vi "Test Panel - Multiple Loops.vi"(7 "Sequence Loop Settings":T4={"Number of Loops"=1, "Delay Between Loops"=0.5} {"Delay Between Loops" format="%#_6ps"}, 8 "Error in":errorcluster, 9 "TDMS Name Mapping":T6={"FGEN Channel Mapping"=[["0", "Chn0"]], "DAQ Channel Mapping"=[["port0/line1", "PA ON"], ["port0/line2", "Gate IN"], ["port0/line3", "Damping"], ["port0/line4", "Rx ON"]], "FGEN Wfm List"=[["Wfm1", "FGEN_Wfm1"], ["Wfm2", "FGEN_Wfm2"]], "DAQ Wfm List"=[["Wfm1", "DAQ_Wfm1"], ["Wfm2", "DAQ_Wfm2"]]}, 10 "Wavefom Sequence":T5={"FGEN Wfm Sequence"=["Wfm1"], "DAQ Wfm Sequence"=["Wfm1"], "Loops"=[1]}, 11 "Resource Settings":T3={"FGEN Resource"="", "DAQmx Resource"="", "TDMS File Path"=path "", "Scope Resource"="", "Scope Config File Path"=path "", "Trigger Delay"=0.0, "Duration"=-1.0, "Fetch Timeout"=5.0} {"Fetch Timeout" format="%#.5ps"; "Duration" format="%#_6ps"; "Trigger Delay" format="%#_gs"}) -> (0 "Error out":errorcluster, 1 "FFT Waveforms (dB)":T8(graph), 2 "FFT Waveforms (Volt RMS)":T8(graph), 3 "Time Domain Waveforms":T8(graph), 4 "All Results Ctrl Refs":T10, 5 "Average FFT (dB)":T8(graph))   [LabVIEW 2025]
uses:
  Live Graph Plotter/Live Graph Plotter.lvclass
  <extravilib>/ChannelInstances/Tag-bool.lvlib
  Typedef/Scope Result Ctrl Refs.ctl
  Typedef/TDMS Name Mapping.ctl
  Typedef/Resource Settings.ctl
panel:
  out "Actual Sample Rates":T1 {"FGEN Sample Rate" format="%#_6pHz"; "DAQ Sample Rate" format="%#_6pHz"; "SCOPE Sample Rate" format="%#_6pHz"}
  in  "Stop":bool
  in  "Tab Control":T2(tab)
  in  "Results":T7(tab)
  in  "Wfm Source - Average FFT (dB)":T9={"Record Start Index (0)"=0, "Record Length (-1)"=-1, "Channel List (All)"=""}
  # "FGEN - Scope - Digital DAQ Test Panel (Multiple Loops)"
  # "Right-click the graph to export waveforms to file"
  # "Then, configure the FGEN and DAQ Sequence accordingly. By default, each step \nonly loops once. You can increase it to more. The number  of records to be captured \nby SCOPE will be total number of loops. You must make sure the number of \nsequence steps and loops are equal. The code doesn't check the consistency."
  # "* Negative duration will keep the original waveform length in the scope settings"
  # "* Make sure the number of elements in each array are match"
  # "This Test Panel can control FGEN and DAQ to generate a sequence of analog and \ndigital waveforms from a TDMS file. While generating, it can also control SCOPE to \ncapture multiple records according to the number of steps in the Waveform \nSequence (FGEN or DAQ).\n\nYou can choose to disable FGEN, DAQ or SCOPE function by leaving thier Resource \nNames blank. \n\nIf FGEN and DAQ are enabled, DAQ will arm the FGEN start trigger before it starts \ngeneration through the PXI backplane (implicit triggering). If only DAQ enabled,\nDAQ will start generation immediately.\n\nBefore start, prepare a TMDS waveform file that matches the TDMS Name Mapping:\n  - For FGEN:\n      - Refer to the FGEN Channel Mapping and FGEN Wfm List.\n      - FGEN will run with the Arbitrary Sequence mode and Single Trigger mode to \n         generate the waveforms in the FGEN Wfm Sequence. \n      - Data will resampled to the highest sample rate among all the FGEN waveforms.\n  - For DAQ:\n     - Refer to the DAQ Channel Mapping and DAQ Wfm List\n     - The waveforms specified in the DAQ Wfm Sequence will be cascaded as one \n        waveform for each channel. \n     - Data will resampled to the highest sample rate among all the DAQ waveforms.\n\nThen, configure the FGEN and DAQ Sequence accordingly. By default, each step \nonly loops once. You can increase it to more. The number  of records to be captured \nby SCOPE will be total number of loops. You must make sure the number of \nsequence steps and loops are equal. The code doesn't check the consistency.  \n\nUse the InstrumentStudio to configure the settings of SCOPE first, and export the \nsettings as .niscopeconfig file. Then, you can use the file to configure the settings\nin this Test Panel."
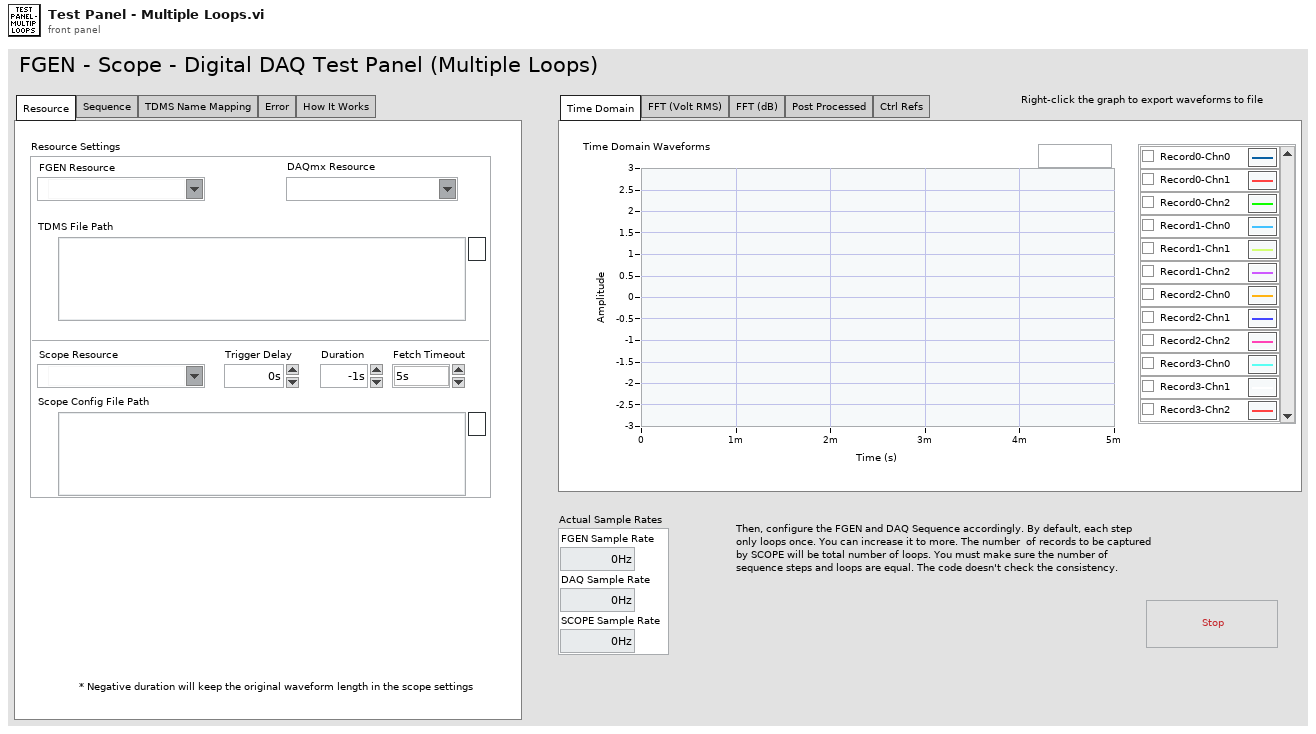
[diagram p1: front panel]
types:
  T1 = cluster{"FGEN Sample Rate":dbl, "DAQ Sample Rate":dbl, "SCOPE Sample Rate":dbl}
  T2 = enum32{"Resource", "Sequence", "TDMS Name Mapping", "Error", "How It Works"}
  T3 = typedef "Resource Settings.ctl" = cluster{"FGEN Resource":refnum<k15>, "DAQmx Resource":tag, "TDMS File Path":path, "Scope Resource":refnum<k15>, "Scope Config File Path":path, "Trigger Delay":dbl, "Duration":dbl, "Fetch Timeout":dbl}
  T4 = cluster{"Number of Loops":u32, "Delay Between Loops":dbl}
  T5 = cluster{"FGEN Wfm Sequence":string[], "DAQ Wfm Sequence":string[], "Loops":i32[]}
  T6 = typedef "TDMS Name Mapping.ctl" = cluster{"FGEN Channel Mapping":string[][], "DAQ Channel Mapping":string[][], "FGEN Wfm List":string[][], "DAQ Wfm List":string[][]}
  T7 = enum32{"Time Domain", "FFT (Volt RMS)", "FFT (dB)", "Post Processed", "Ctrl Refs"}
  T8 = cluster{"relativeInitialX":dbl, "xIncrement":dbl, "wfm":dbl[]}[]
  T9 = cluster{"Record Start Index (0)":i32, "Record Length (-1)":i32, "Channel List (All)":string}
  T10 = cluster{"Time Waveforms Graph Ref":refnum<class "Live Graph Plotter.lvclass">, "FFT Volt RMS Graph Ref":refnum<class "Live Graph Plotter.lvclass">, "FFT dB Graph Ref":refnum<class "Live Graph Plotter.lvclass">, "Live Graph Plotter out":refnum<class "Live Graph Plotter.lvclass">}
  T11 = typedef "Scope Result Ctrl Refs.ctl" = cluster{"Time Waveforms Graph Ref":refnum<class "Live Graph Plotter.lvclass">, "FFT Volt RMS Graph Ref":refnum<class "Live Graph Plotter.lvclass">, "FFT dB Graph Ref":refnum<class "Live Graph Plotter.lvclass">}
  T12 = typedef "Test Panel State Data.ctl" = cluster{"FGEN Resource":refnum<k15>, "DAQmx Tasks Session":cluster{"DO Task":refnum<k21>, "Ctr0 Task":refnum<k21>}, "Scope Resource":refnum<k15>, "FGEN Enabled?":bool, "DAQ Enabled?":bool, "Scope Enabled?":bool, "Max Total FGEN Wfm Duration (s)":dbl, "FGEN-DAQ Routing":cluster{"FGEN Start Trigger":string, "DAQ Trig Line":string}, "Scope Recording Settings":T13}
  T13 = typedef "Scope Recording Settings.ctl" = cluster{"Number of Records":i32, "Channels Per Record":i32, "Plot Names":string[][], "Fetch Timeout":dbl, "Channel List":string}
  T14 = typedef "Tag-bool.lvlib/))Channel.ctl" = refnum<queue>
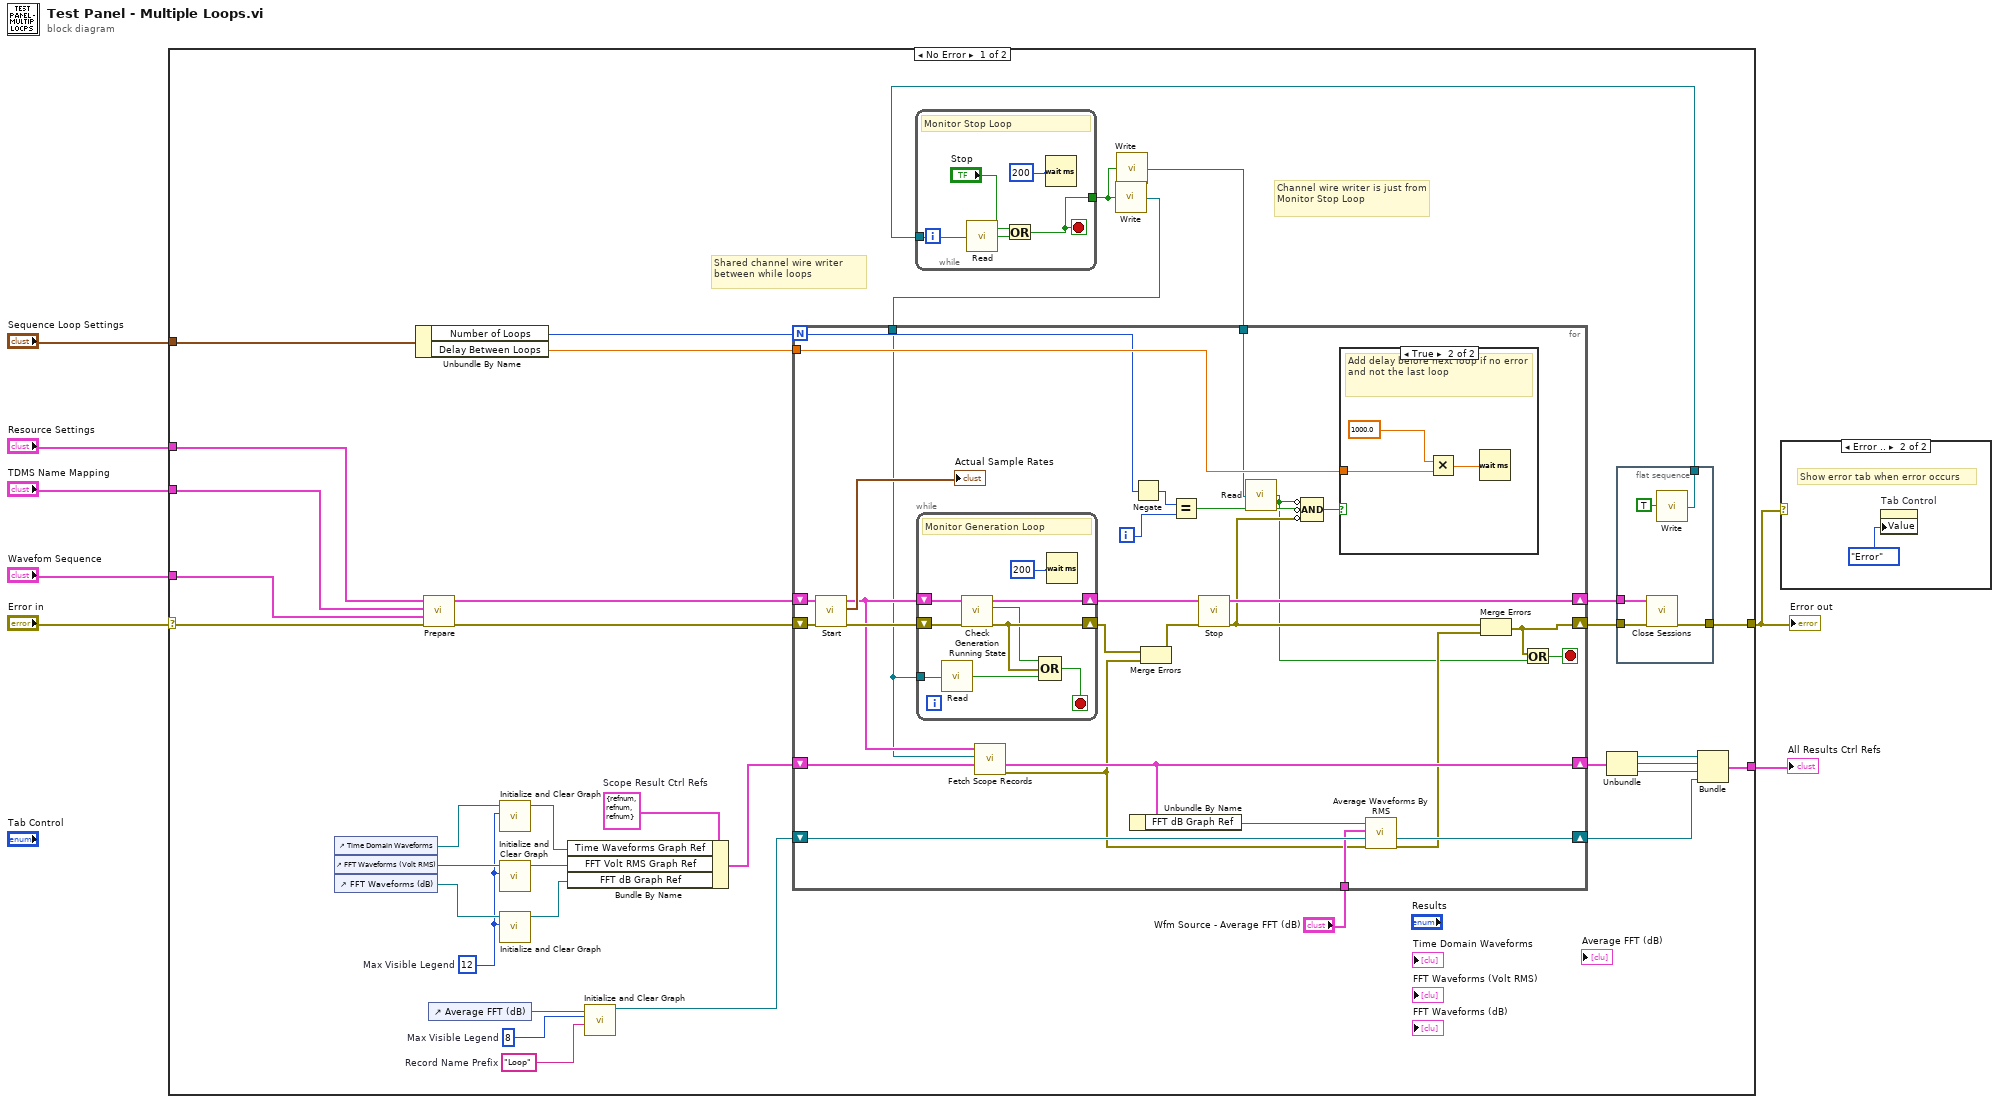
[diagram p0: block diagram]
diagram:
  n1 = case shown="No Error" "Error in" {
    selector: "Error in" -> [w40 w95]
    tunnel: [w37 w95] -> w4
    tunnel: "Resource Settings" -> [w43 _]
    tunnel: "TDMS Name Mapping" -> [w42 _]
    tunnel: "Wavefom Sequence" -> [w41 _]
    tunnel: "Sequence Loop Settings" -> [w25 _]
    tunnel: [w8 _] -> w1
    frame No Error {
      w18 = "Loop"  # Record Name Prefix
      w21 = 8  # Max Visible Legend
      w28 = 12  # Max Visible Legend
      w36 = T11 {"Time Waveforms Graph Ref"=refnum, "FFT Volt RMS Graph Ref"=refnum, "FFT dB Graph Ref"=refnum}  # Scope Result Ctrl Refs
      # "Channel wire writer is just from Monitor Stop Loop"
      # "Shared channel wire writer between while loops"
      n2 = control-ref of="Time Domain Waveforms"() -> (w34:refnum<vi>)
      n3 = control-ref of="FFT Waveforms (Volt RMS)"() -> (w33:refnum<vi>)
      n4 = control-ref of="FFT Waveforms (dB)"() -> (w29:refnum<vi>)
      n5 = Unbundle By Name(w25) -> ("Number of Loops"=w24:u32, "Delay Between Loops"=w23:dbl)
      n6 = call "Prepare.vi"("error in (no error)"=w40, "Wavefom Sequence"=w41, "TDMS Name Mapping"=w42, "Resource Settings"=w43) -> ("error out"=w39:errorcluster, "Panel State Data Out"=w38:T12)  [unwired: 6 in]
      n7 = control-ref of="Average FFT (dB)"() -> (w22:refnum<vi>)
      n8 = call "Initialize and Clear Graph.vi"("Max Visible Legend"=w28, "WaveformGraph Ref"=w34) -> ("Live Graph Plotter out"=w32:refnum<class "Live Graph Plotter.lvclass">)  [unwired: 8 in, 1 out]
      n9 = call "Initialize and Clear Graph.vi"("Max Visible Legend"=w28, "WaveformGraph Ref"=w33) -> ("Live Graph Plotter out"=w31:refnum<class "Live Graph Plotter.lvclass">)  [unwired: 8 in, 1 out]
      n10 = call "Initialize and Clear Graph.vi"("Max Visible Legend"=w28, "WaveformGraph Ref"=w29) -> ("Live Graph Plotter out"=w30:refnum<class "Live Graph Plotter.lvclass">)  [unwired: 8 in, 1 out]
      n11 = Bundle By Name(cluster=w36, "Time Waveforms Graph Ref"=w32, "FFT Volt RMS Graph Ref"=w31, "FFT dB Graph Ref"=w30) -> (w35:T11)
      n12 = call "Initialize and Clear Graph.vi"("Record Name Prefix"=w18, "Max Visible Legend"=w21, "WaveformGraph Ref"=w22) -> ("Live Graph Plotter out"=w20:refnum<class "Live Graph Plotter.lvclass">)  [unwired: 7 in, 1 out]
      n13 = while {
        tunnel: [w92] -> w15
        tunnel: w17 -> [w91]
        stop <- w92 stop-if-true
        # "Monitor Stop Loop"
        n14 = call <extravilib>:"Read.vi"("channel"=w91) -> ("element"=w90:bool)  [unwired: 1 in, 1 out]
        n15 = Or(x="Stop", y=w90) -> (x .or. y?=w92:bool)
        n16 = Wait (ms)(milliseconds to wait=u32 200) -> ()  [unwired: 1 out]
      }
      n17 = call <extravilib>:"Write.vi"("element"=w15) -> ("channel"=w16:T14)  [unwired: 1 out]
      n18 = call <extravilib>:"Write.vi"("element"=w15) -> ("channel"=w14:T14)  [unwired: 1 out]
      n19 = for {
        N: w24 -> [w65]
        shift-right: [w51] -> w27
        shift-left: w39 -> [w55]
        shift-right: [w69] -> w26
        shift-left: w38 -> [w77]
        tunnel: w23 -> [w68]
        shift-right: [w60] -> w13
        shift-left: w35 -> [w71]
        tunnel: "Wfm Source - Average FFT (dB)" -> [w61]
        shift-right: [w58] -> w9
        shift-left: w20 -> [w62]
        tunnel: w16 -> [w54]
        tunnel: w14 -> [w52]
        i -> [w64]
        stop <- w49 stop-if-true
        n20 = call "Start.vi"("error in (no error)"=w55, "Panel State Data In"=w77) -> ("error out"=w75:errorcluster, "Actual Sample Rates"=→"Actual Sample Rates":T1, "Panel State Data Out"=w74:T12)  [unwired: 7 in]
        n21 = while {
          shift-right: [w86] -> w73
          shift-left: w75 -> [w89]
          shift-right: [w85] -> w70
          shift-left: w74 -> [w88]
          tunnel: w54 -> [w82]
          stop <- w87 stop-if-true
          # "Monitor Generation Loop"
          n22 = call <extravilib>:"Read.vi"("channel"=w82) -> ("element"=w81:bool)  [unwired: 1 in, 1 out]
          n23 = call "Check Generation Running State.vi"("error in (no error)"=w89, "Panel State Data In"=w88) -> ("error out"=w86:errorcluster, "Is Done?"=w83:bool, "Panel State Data Out"=w85:T12)  [unwired: 7 in]
          n24 = Compound Arithmetic op=OR(w83, w86, w81) -> (w87:bool)
          n25 = Wait (ms)(milliseconds to wait=u32 200) -> ()  [unwired: 1 out]
        }
        n26 = call "Fetch Scope Records.vi"("Scope Result Ctrl Refs In"=w71, "Stop Channel"=w54, "Panel State Data In"=w74) -> ("error out"=w53:errorcluster, "Scope Result Ctrl Refs Out"=w60:T11)  [unwired: 6 in, 1 out]
        n27 = Unbundle By Name(w60) -> ("FFT dB Graph Ref"=w59:refnum<class "Live Graph Plotter.lvclass">)
        n28 = Negate(x=w65) -> (-x=w66:i32)
        n29 = Merge Errors(w73, w53) -> (w72:errorcluster)
        n30 = Equal?(x=w66, y=w64) -> (x = y?=w63:bool)
        n31 = call "Stop.vi"("error in (no error)"=w72, "Panel State Data In"=w70) -> ("error out"=w56:errorcluster, "Panel State Data Out"=w69:T12)  [unwired: 8 in]
        n32 = call <extravilib>:"Read.vi"("channel"=w52) -> ("element"=w50:bool)  [unwired: 1 in, 1 out]
        n33 = Compound Arithmetic op=AND(invert w50, invert w63, invert w56) -> (w67:bool)
        n34 = case shown="True" w67 {
          tunnel: w68 -> [_ w80]
          frame False {
          }
          frame True {
            # "Add delay before next loop if no error and not the last loop"
            n35 = Multiply(x=1000.0, y=w80) -> (x*y=w79:dbl)
            n36 = Wait (ms)(milliseconds to wait=w79) -> ()  [unwired: 1 out]
          }
        }
        n37 = call "Average Waveforms By RMS.vi"("error in"=w53, "Result Live Graph Plotter in"=w62, "Waveforms Selection"=w61, "Original Live Graph Plotter in"=w59) -> ("error out"=w57:errorcluster, "Result Live Graph Plotter out"=w58:refnum<class "Live Graph Plotter.lvclass">)  [unwired: 6 in]
        n38 = Merge Errors(w56, w57) -> (w51:errorcluster)
        n39 = Or(x=w51, y=w50) -> (x .or. y?=w49:bool)
      }
      n40 = Unbundle(w13) -> ("Time Waveforms Graph Ref"=w12:refnum<class "Live Graph Plotter.lvclass">, "FFT Volt RMS Graph Ref"=w11:refnum<class "Live Graph Plotter.lvclass">, "FFT dB Graph Ref"=w10:refnum<class "Live Graph Plotter.lvclass">)
      n41 = flat-sequence {
        tunnel: [w48] -> w37
        tunnel: w27 -> [w47]
        tunnel: w26 -> [w46]
        tunnel: [w44] -> w17
        frame #0 {
          n42 = call "Close Sessions.vi"("error in (no error)"=w47, "Panel State Data In"=w46) -> ("error out"=w48:errorcluster)  [unwired: 8 in, 1 out]
          n43 = call <extravilib>:"Write.vi"("element"=TRUE) -> ("channel"=w44:T14)  [unwired: 1 out]
        }
      }
      n44 = Bundle("Time Waveforms Graph Ref"=w12, "FFT Volt RMS Graph Ref"=w11, "FFT dB Graph Ref"=w10, "Live Graph Plotter out"=w9) -> (w8:T10)  [unwired: 1 in]
    }
    frame Error {
    }
  }
  "Error out" <- w4
  "All Results Ctrl Refs" <- w1
  n45 = case shown="Error .." w4 {
    frame No Error {
    }
    frame Error {
      # "Show error tab when error occurs"
      n46 = property on="Tab Control" class="TabCtl (strict)"("Value"=T2."Error" ("Tab Control")) -> ()  [unwired: 2 in, 2 out]
    }
  }
